vi "SW_Get_1D_Array_normalize.vi"(2 "Error In":errorcluster, 4 "1D array":dbl[](array[numeric])) -> (0 "Error Out":errorcluster, 1 "Normalized 1D array":dbl[](array[numeric]))   [LabVIEW 2016]
panel:
  in  "N points":u16=300
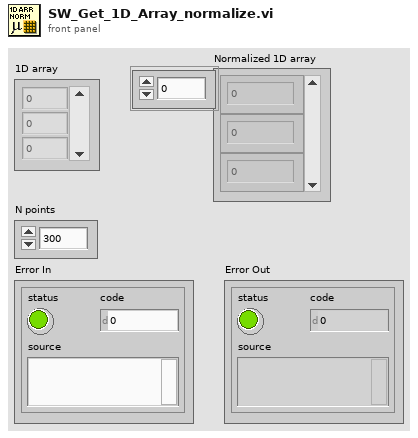
[diagram p1: front panel]
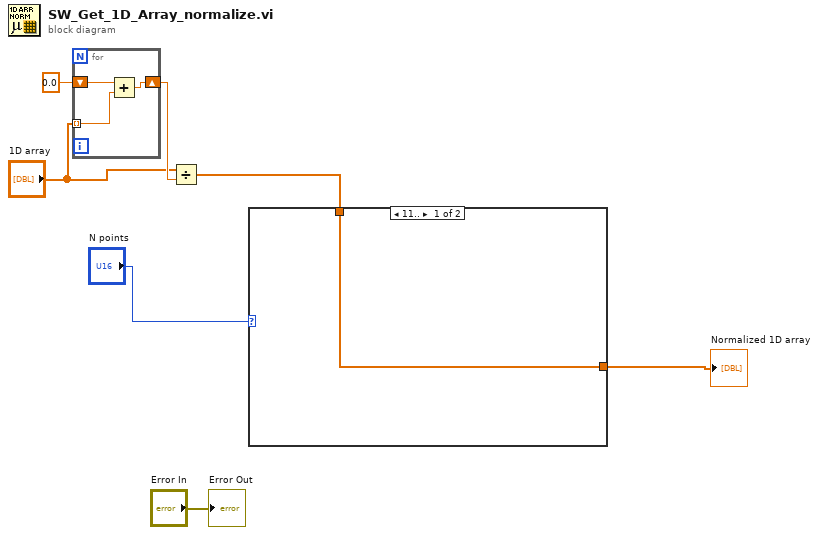
[diagram p0: block diagram]
diagram:
  n1 = for {
    tunnel: "1D array" -> [w10] mode=indexing
    shift-right: [w9] -> w6
    shift-left: 0.0 -> [w8]
    n2 = Add(x=w8, y=w10) -> (x+y=w9:dbl)
  }
  n3 = Divide(x="1D array", y=w6) -> (x/y=w2:dbl[])
  n4 = case shown="11.." "N points" {
    tunnel: [w11 w12] -> w3
    tunnel: w2 -> [w11 w12]
    frame 11.. {
    }
    frame 0..10, Default {
    }
  }
  "Normalized 1D array" <- w3
  "Error Out" <- "Error In"
